vi "NF WF1973_74 SRE.vi"(6 "Read(F)":bool, 8 "error in (no error)":errorcluster caption="Error IN", 10 "SRE(0)":i32(knob) min=0 max=254 step=1 scale=0.0..254.0, 11 "VISAsession":refnum<visa-resource-name>) -> (0 "error out":errorcluster caption="Error OUT", 2 "Query SRE":i32=999, 3 "CopyVISAsession":refnum<visa-resource-name>)   [LabVIEW 2010]
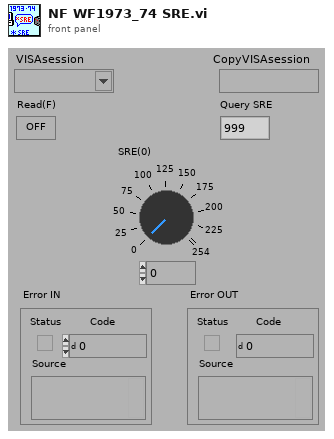
[diagram p1: front panel]
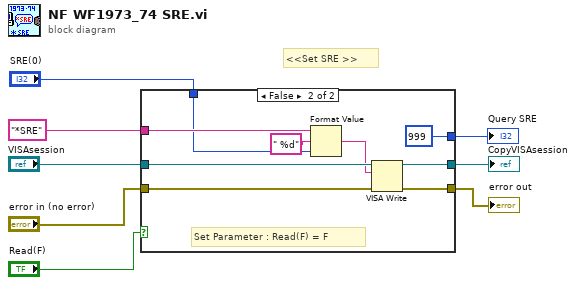
[diagram p0: block diagram]
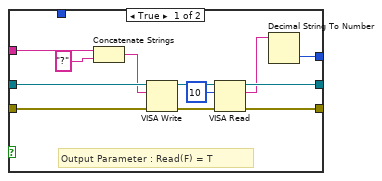
[diagram p2: hidden frame]
diagram:
  # "<<Set SRE >>"
  n1 = case shown="FALSE" "Read(F)" {
    tunnel: "VISAsession" -> [w20 w29]
    tunnel: [w11 w26] -> w7
    tunnel: [w17 w27] -> w6
    tunnel: "error in (no error)" -> [w16 w28]
    tunnel: "*SRE" ("文字列") -> [w14 w25]
    tunnel: "SRE(0)" -> [_ w22]
    tunnel: [w9 999] -> w1
    frame True {
      # "Output Parameter : Read(F) = T"
      n2 = Concatenate Strings(w14, "?" ("形式文字列")) -> (w12:string)
      n3 = VISA Write(VISA resource name=w20, write buffer=w12, error in (no error)=w16) -> (VISA resource name out=w18:refnum<visa-resource-name>, error out=w19:errorcluster)  [unwired: 1 out]
      n4 = VISA Read(VISA resource name=w18, byte count=u32 10 ("バイトカウント（0）"), error in (no error)=w19) -> (VISA resource name out=w11:refnum<visa-resource-name>, read buffer=w10:string, error out=w17:errorcluster)  [unwired: 1 out]
      n5 = Decimal String To Number(string=w10) -> (number=w9:i32)  [unwired: 2 in, 1 out]
    }
    frame False {
      # "Set Parameter : Read(F) = F"
      n6 = Format Value(string ("")=w25, format string=" %d" ("形式文字列"), value (0)=w22) -> (output string=w23:string)
      n7 = VISA Write(VISA resource name=w29, write buffer=w23, error in (no error)=w28) -> (VISA resource name out=w26:refnum<visa-resource-name>, error out=w27:errorcluster)  [unwired: 1 out]
    }
  }
  "error out" <- w6
  "CopyVISAsession" <- w7
  "Query SRE" <- w1
